vi "c Spark Clear Faults.vi"(8 "error in (no error)":errorcluster, 11 "handle":T1) -> (0 "error out":errorcluster, 2 "function return":T2, 3 "handle":T1)   [LabVIEW 2023, in "REVLibDriver.lvlib"]
doc: "c_REVLib_ErrorCode c_Spark_ClearFaults(c_Spark_handle handle);"
uses:
  REVLibDriver.lvlib
  REVLibDriver.dll
  <vilib>/Custom Controls/c_Spark_handle.ctl
  subvi/RevLibError.ctl
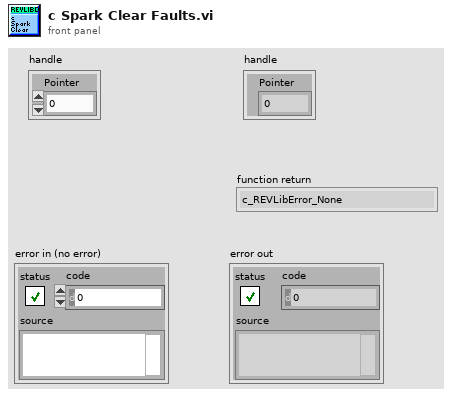
[diagram p1: front panel]
types:
  T1 = typedef "REVLibDriver.lvlib/c_Spark_handle.ctl" = cluster{"Pointer":u32}
  T2 = typedef "REVLibDriver.lvlib/RevLibError.ctl" = enum16{"c_REVLibError_None", "c_REVLibError_General", "c_REVLibError_CANTimeout", "c_REVLibError_NotImplemented", "c_REVLibError_HAL", "c_REVLibError_CantFindFirmware", "c_REVLibError_FirmwareTooOld", "c_REVLibError_FirmwareTooNew", "c_REVLibError_ParamInvalidID", "c_REVLibError_ParamMismatchType", "c_REVLibError_ParamAccessMode", "c_REVLibError_ParamInvalid", "c_REVLibError_ParamNotImplementedDeprecated", "c_REVLibError_FollowConfigMismatch", "c_REVLibError_Invalid", "c_REVLibError_SetpointOutOfRange", "c_REVLibError_Unknown", "c_REVLibError_CANDisconnected", "c_REVLibError_DuplicateCANId", "c_REVLibError_InvalidCANId", "c_REVLibError_SparkMaxDataPortAlreadyConfiguredDifferently", "c_REVLibError_SparkFlexBrushedWithoutDock", "c_REVLibError_NumCodes"}
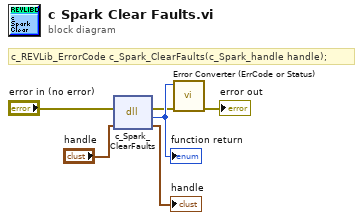
[diagram p0: block diagram]
diagram:
  # "c_REVLib_ErrorCode c_Spark_ClearFaults(c_Spark_handle handle);"
  n1 = dll-call lib="REVLibDriver.*" fn="c_Spark_ClearFaults"(error in="error in (no error)", "handle"="handle") -> (error out=w2:errorcluster, "return type"=w6:u32, "handle"=→"handle":T1)  [unwired: 2 in, 1 out]
  "function return" <- w6
  n2 = call "Error Converter (ErrCode or Status).vi"("error in (no error)"=w2, "error code"=w6) -> ("error out"=→"error out":errorcluster)  [unwired: 9 in]
